vi "2dArrayToNx1Array.vi"(11 "2D Array":dbl[][](array[numeric])) -> (3 "nx1 Array":dbl[][](array[numeric]))   [LabVIEW 2016]
doc: "Transform mxn array to (m*n)x1 array."
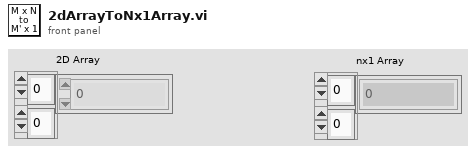
[diagram p1: front panel]
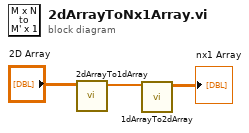
[diagram p0: block diagram]
diagram:
  n1 = call "2dArrayTo1dArray.vi"("2D Array"="2D Array") -> ("1D Array"=w2:dbl[])  [unwired: 10 in]
  n2 = call "1dArrayTo2dArray.vi"("1D Array"=w2) -> ("2D Array"=→"nx1 Array":dbl[][])  [unwired: 10 in]
